vi "clear.vi"(8 "error in (no error)":errorcluster, 11 "State in":refnum<class "ElectrometerState.lvclass">) -> (0 "error out":errorcluster, 3 "State out":refnum<class "ElectrometerState.lvclass">)   [LabVIEW 2016, in "ElectrometerState.lvclass"]
uses:
  ElectrometerState.lvclass
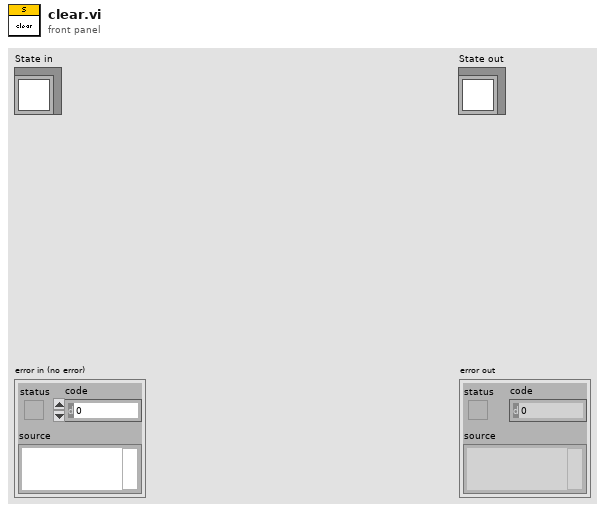
[diagram p1: front panel]
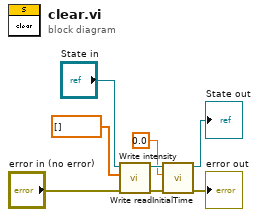
[diagram p0: block diagram]
diagram:
  n1 = call-dynamic "Write intensity.vi"("error in (no error)"="error in (no error)", "intensity"=dbl[] [], "State in"="State in") -> ("error out"=w4:errorcluster, "State out"=w7:refnum<class "ElectrometerState.lvclass">)  [unwired: 7 in]
  n2 = call-dynamic "Write readInitialTime.vi"("error in (no error)"=w4, "readInitialTime"=0.0, "State in"=w7) -> ("error out"=→"error out":errorcluster, "State out"=→"State out":refnum<class "ElectrometerState.lvclass">)  [unwired: 7 in]
